vi "Get BufferLastReadsDBL.vi"(11 "Thermometer DAQmx RTD Cont CFG in":refnum<class "Thermometer DAQmx RTD Cont CFG.lvclass">) -> (2 "BufferLastReadsDBL.lvclass":refnum<class "BufferLastReadsDBL.lvclass">, 3 "Thermometer DAQmx RTD Cont CFG out":refnum<class "Thermometer DAQmx RTD Cont CFG.lvclass">)   [LabVIEW 2024, in "Thermometer DAQmx RTD Cont CFG.lvclass"]
uses:
  Thermometer DAQmx RTD Cont CFG.lvclass
  Thermometer DAQmx RTD Cont CFG.lvclass/Thermometer DAQmx RTD Cont CFG.ctl
  Buffers/BufferLastReadingsDBL/BufferLastReadsDBL.lvclass
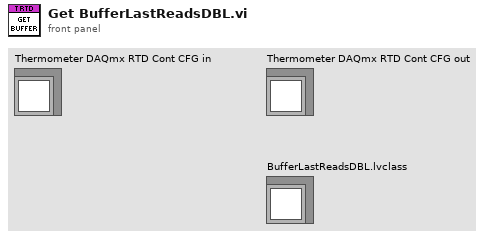
[diagram p1: front panel]
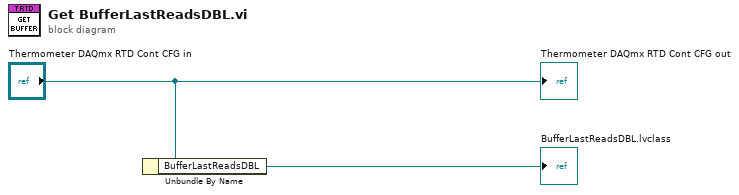
[diagram p0: block diagram]
diagram:
  n1 = Unbundle By Name("Thermometer DAQmx RTD Cont CFG in") -> ("BufferLastReadsDBL"=→"BufferLastReadsDBL.lvclass":refnum<class "BufferLastReadsDBL.lvclass">)
  "Thermometer DAQmx RTD Cont CFG out" <- "Thermometer DAQmx RTD Cont CFG in"
